vi "test Simple Blob.vi"(8 "error in (no error)":errorcluster, 11 "TestCase in":refnum<class "Test_Blob.lvclass">) -> (0 "error out":errorcluster, 3 "TestCase out":refnum<class "Test_Blob.lvclass">)   [LabVIEW 2015, in "Test_Blob.lvclass"]
uses:
  Test_Blob.lvclass
  Blob Storage/Blob Type.ctl
  Global Parameters.vi
  Core/Session/Session.lvclass
  Blob Storage/NI_Azure_Blob.lvlib
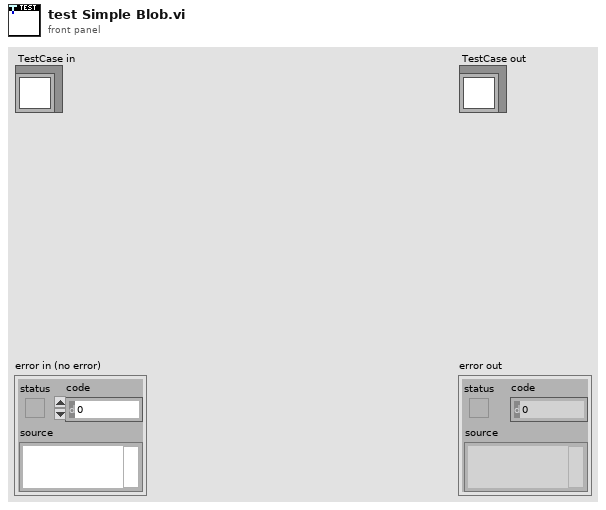
[diagram p1: front panel]
types:
  T1 = typedef "NI_Azure_Blob.lvlib/Blob Type.ctl" = enum16{"BlockBlob", "PageBlob", "AppendBlob"}
  T2 = typedef "NI_Azure_Core.lvlib/Session.lvclass/Azure Credentials.ctl" = cluster{"Storage Account Name":string, "Access Key":string}
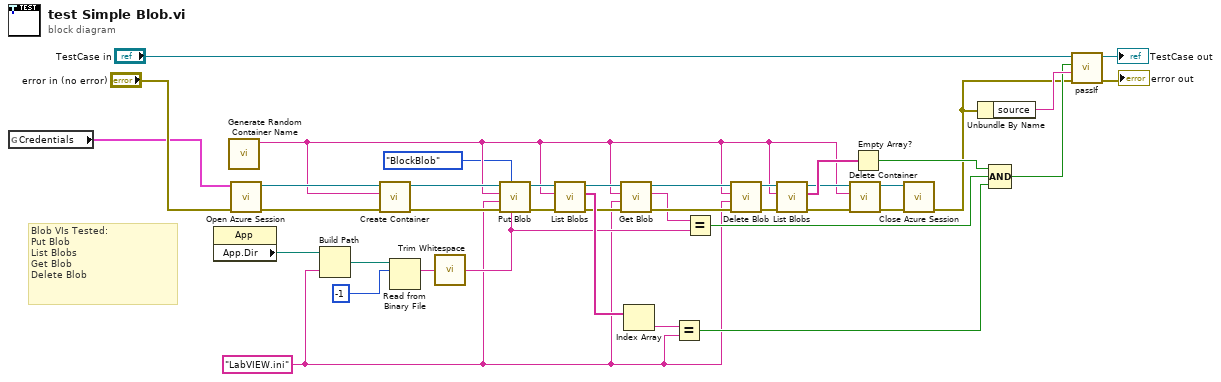
[diagram p0: block diagram]
diagram:
  w6 = "LabVIEW.ini"
  # "Blob VIs Tested:\nPut Blob\nList Blobs\nGet Blob\nDelete Blob"
  n1 = global read "Global Parameters.vi" "Credentials"() -> (w11:T2)
  n2 = property class="App"() -> ("App.Dir"=w35:path)  [unwired: 2 in, 2 out]
  n3 = call "Generate Random Container Name.vi"() -> ("Random Container Name"=w5:string)  [unwired: 11 in]
  n4 = call "Open Azure Session.vi"("error in (no error)"="error in (no error)", "Credentials"=w11) -> ("error out"=w12:errorcluster, "Azure Session"=w8:refnum<class "Session.lvclass">)  [unwired: 8 in]
  n5 = Build Path(base path=w35, name or relative path=w6) -> (appended path=w34:path)
  n6 = call "Create Container.vi"("error in (no error)"=w12, "Container"=w5, "Azure Session in"=w8) -> ("error out"=w32:errorcluster, "Azure Session out"=w31:refnum<class "Session.lvclass">)  [unwired: 7 in]
  n7 = Read from Binary File(10:-1 ("count (1)"), 11:w34) -> (2:w25:string)  [unwired: 4 in, 3 out]
  n8 = call <vilib>:"Trim Whitespace.vi"("string"=w25) -> ("trimmed string"=w7:string)  [unwired: 1 in]
  n9 = call "Put Blob.vi"("Blob Content"=w7, "Blob type"=Blob_Type."BlockBlob", "error in (no error)"=w32, "Blob"=w6, "Container"=w5, "Azure Session in"=w31) -> ("error out"=w30:errorcluster, "Azure Session out"=w29:refnum<class "Session.lvclass">)  [unwired: 4 in]
  n10 = call "List Blobs.vi"("error in (no error)"=w30, "Container"=w5, "Azure Session in"=w29) -> ("error out"=w27:errorcluster, "Blobs"=w28:string[], "Azure Session out"=w26:refnum<class "Session.lvclass">)  [unwired: 6 in]
  n11 = call "Get Blob.vi"("error in (no error)"=w27, "Blob"=w6, "Container"=w5, "Azure Session in"=w26) -> ("error out"=w23:errorcluster, "Blob Content"=w4:string, "Azure Session out"=w22:refnum<class "Session.lvclass">)  [unwired: 5 in]
  n12 = Index Array(array=w28) -> (element=w21:string)  [unwired: 1 in]
  n13 = Equal?(x=w21, y=w6) -> (x = y?=w20:bool)
  n14 = Equal?(x=w4, y=w7) -> (x = y?=w24:bool)
  n15 = call "Delete Blob.vi"("error in (no error)"=w23, "Blob"=w6, "Container"=w5, "Azure Session in"=w22) -> ("error out"=w19:errorcluster, "Azure Session out"=w18:refnum<class "Session.lvclass">)  [unwired: 6 in]
  n16 = call "List Blobs.vi"("error in (no error)"=w19, "Container"=w5, "Azure Session in"=w18) -> ("error out"=w15:errorcluster, "Blobs"=w17:string[], "Azure Session out"=w14:refnum<class "Session.lvclass">)  [unwired: 6 in]
  n17 = call "Delete Container.vi"("error in (no error)"=w15, "Container"=w5, "Azure Session in"=w14) -> ("error out"=w10:errorcluster, "Azure Session out"=w1:refnum<class "Session.lvclass">)  [unwired: 7 in]
  n18 = Empty Array?(array=w17) -> (empty?=w16:bool)
  n19 = call "Close Azure Session.vi"("error in (no error)"=w10, "Azure Session"=w1) -> ("error out"=w2:errorcluster)  [unwired: 9 in]
  n20 = Unbundle By Name(w2) -> ("source"=w36:string)
  n21 = Compound Arithmetic op=AND(w16, w24, w20) -> (w9:bool)
  n22 = call-dynamic "passIf.vi"("error in (no error)"=w2, "message (\"\")"=w36, "pass"=w9, "TestCase in"="TestCase in") -> ("error out"=→"error out":errorcluster, "TestCase out"=→"TestCase out":refnum<class "Test_Blob.lvclass">)  [unwired: 6 in]
